vi "SCCSup IsSCCDisabled.vi"(8 "error in (no error)":errorcluster) -> (0 "error out":errorcluster, 2 "SCC disabled?":bool, 5 "initialized?":bool)   [LabVIEW 2020]
uses:
  <vilib>/SourceControl/sccconnsrv/SCC_ConnSrv Op FGEvent.ctl
  <vilib>/SourceControl/sccconnsrv/NI_SCC_ConnSrv.lvlib
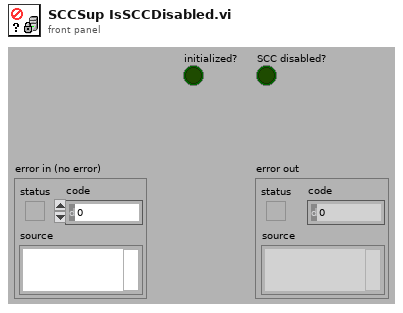
[diagram p1: front panel]
types:
  T1 = typedef "NI_SCC_ConnSrv.lvlib/SCC_ConnSrv Op FGEvent.ctl" = enum16{"read", "write"}
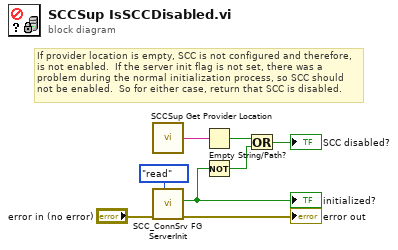
[diagram p0: block diagram]
diagram:
  # "If provider location is empty, SCC is not configured and therefore, is not enabled.  If the server init flag is not set, there was a problem during the normal initialization process, so SCC should not be enabled.  So for either case, return that SCC is disabled."
  n1 = call <vilib>:"SCCSup Get Provider Location.vi"() -> ("provider location"=w5:string)  [unwired: 6 in]
  n2 = call <vilib>:"SCC_ConnSrv FG ServerInit.vi"("FG operation"=SCC_ConnSrv_Op_FGEvent."read", "error in (no error)"="error in (no error)") -> ("error out"=→"error out":errorcluster, "init flag out"=w1:bool)  [unwired: 8 in]
  "initialized?" <- w1
  n3 = Empty String/Path?(string/path=w5) -> (empty?=w7:bool)
  n4 = Not(x=w1) -> (.not. x?=w6:bool)
  n5 = Or(x=w7, y=w6) -> (x .or. y?=→"SCC disabled?":bool)
